vi "Find_rotation_and_offset.vi"(8 "Target 1":dbl[](array[numeric]), 9 "Target 0":dbl[](array[numeric]), 10 "Ref 1":dbl[](array[numeric]), 11 "Ref 0":dbl[](array[numeric])) -> (3 "Transform":T1)   [LabVIEW 2019]
panel:
  out "dqy":dbl
  out "dqx":dbl
  out "dpy":dbl
  out "dpx":dbl
  out "cqx":dbl
  out "cqy":dbl
  out "cpx":dbl
  out "cpy":dbl
  in  "Transform model":T1
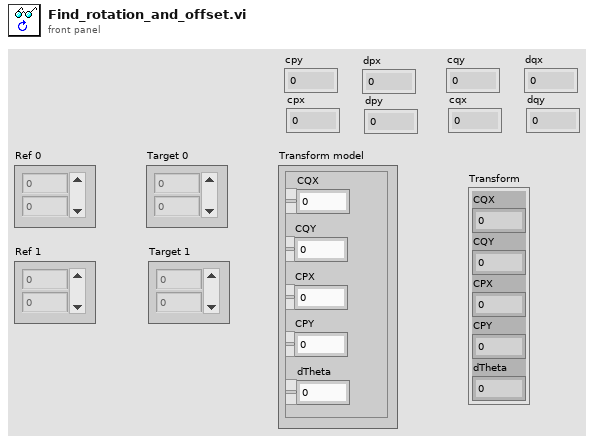
[diagram p1: front panel]
types:
  T1 = cluster{"CQX":dbl, "CQY":dbl, "CPX":dbl, "CPY":dbl, "dTheta":dbl}
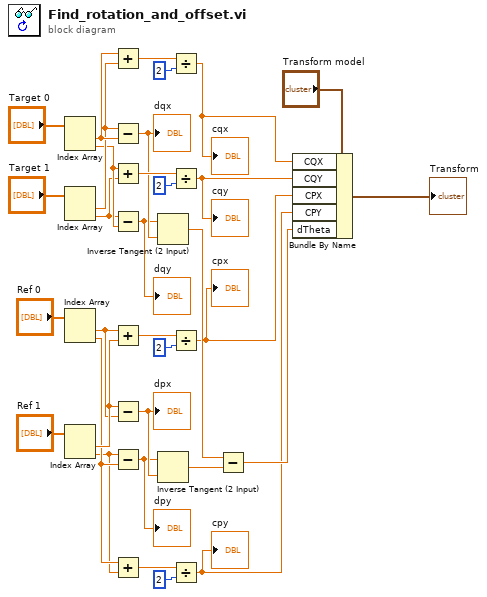
[diagram p0: block diagram]
diagram:
  n1 = Index Array(array="Target 0") -> (element #1=w17:dbl, element #2=w15:dbl)  [unwired: 2 in]
  n2 = Index Array(array="Target 1") -> (element #1=w16:dbl, element #2=w14:dbl)  [unwired: 2 in]
  n3 = Index Array(array="Ref 0") -> (element #1=w20:dbl, element #2=w19:dbl)  [unwired: 2 in]
  n4 = Index Array(array="Ref 1") -> (element #1=w21:dbl, element #2=w18:dbl)  [unwired: 2 in]
  n5 = Add(x=w17, y=w16) -> (x+y=w25:dbl)
  n6 = Subtract(x=w16, y=w17) -> (x-y=w13:dbl)
  "dqx" <- w13
  n7 = Add(x=w15, y=w14) -> (x+y=w26:dbl)
  n8 = Subtract(x=w14, y=w15) -> (x-y=w12:dbl)
  "dqy" <- w12
  n9 = Add(x=w20, y=w21) -> (x+y=w29:dbl)
  n10 = Subtract(x=w21, y=w20) -> (x-y=w11:dbl)
  "dpx" <- w11
  n11 = Subtract(x=w18, y=w19) -> (x-y=w10:dbl)
  "dpy" <- w10
  n12 = Add(x=w19, y=w18) -> (x+y=w30:dbl)
  n13 = Inverse Tangent (2 Input)(1:w13, 2:w12) -> (0:w9:dbl)
  n14 = Inverse Tangent (2 Input)(1:w11, 2:w10) -> (0:w8:dbl)
  n15 = Divide(x=w25, y=2) -> (x/y=w5:dbl)
  "cqx" <- w5
  n16 = Divide(x=w26, y=2) -> (x/y=w4:dbl)
  "cqy" <- w4
  n17 = Divide(x=w29, y=2) -> (x/y=w3:dbl)
  "cpx" <- w3
  n18 = Divide(x=w30, y=2) -> (x/y=w2:dbl)
  "cpy" <- w2
  n19 = Subtract(x=w9, y=w8) -> (x-y=w6:dbl)
  n20 = Bundle By Name(cluster="Transform model", "CQX"=w5, "CQY"=w4, "CPX"=w3, "CPY"=w2, "dTheta"=w6) -> (→"Transform":T1)
